vi "Copy (File).vi"(8 "error in (no error)":errorcluster, 9 "table":string, 10 "Path to spreadsheet":path, 11 "Data.PGSQL":refnum<class "LV-Data.PGSQL.lvclass">) -> (0 "error out":errorcluster, 3 "Data.PGSQL out":refnum<class "LV-Data.PGSQL.lvclass">)   [LabVIEW 2019, in "LV-Data.PGSQL.lvclass"]
uses:
  LV-Data.PGSQL.lvclass
  <vilib>/JDP Science/PostgreSQL Library/Connection/PQ Connection.lvclass
  LV-Data.PGSQL.lvclass/LV-Data.PGSQL.ctl
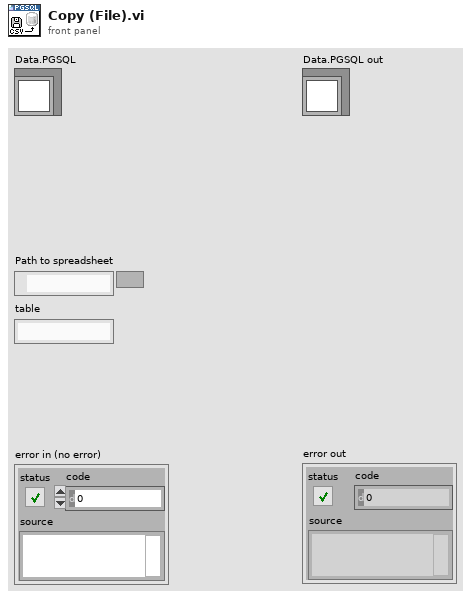
[diagram p1: front panel]
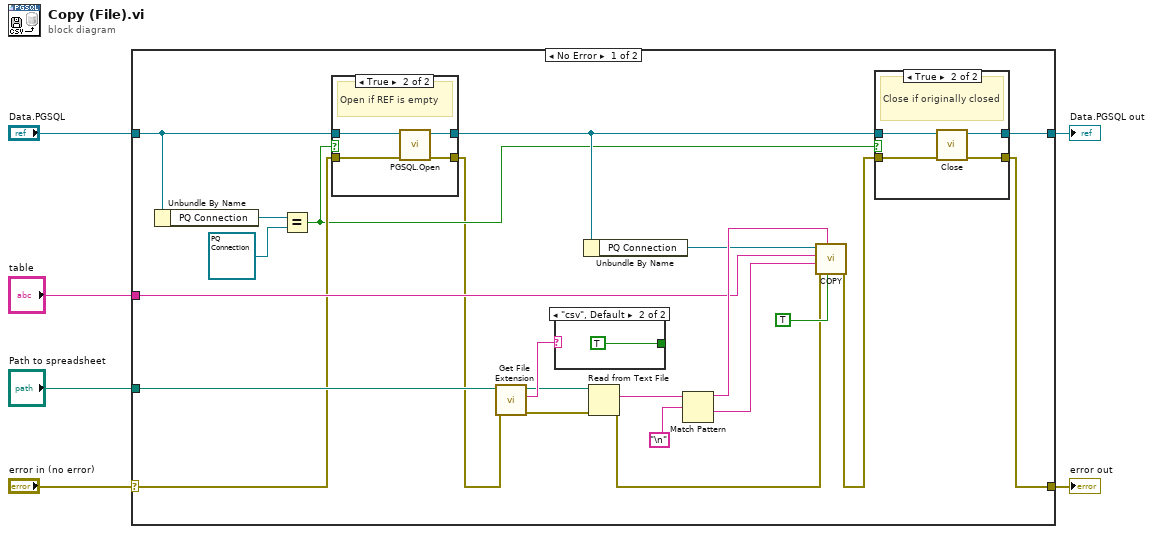
[diagram p0: block diagram]
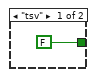
[diagram p3: hidden frame]
diagram:
  n1 = case shown="No Error" "error in (no error)" {
    selector: "error in (no error)" -> [w9 w44]
    tunnel: "table" -> [w17 _]
    tunnel: "Path to spreadsheet" -> [w23 _]
    tunnel: "Data.PGSQL" -> [w10 w43]
    tunnel: [w15 w44] -> w3
    tunnel: [w16 w43] -> w1
    frame No Error {
      n2 = Unbundle By Name(w10) -> ("PQ Connection"=w12:refnum<class "PQ Connection.lvclass">)
      n3 = Equal?(x=w12, y=refnum<class "PQ Connection.lvclass"> refnum ("PQ Connection")) -> (x = y?=w8:bool)
      n4 = case shown="True" w8 {
        tunnel: w10 -> [w29 w32]
        tunnel: [w30 w34] -> w7
        tunnel: w9 -> [w30 w33]
        tunnel: [w29 w31] -> w11
        frame False {
        }
        frame True {
          # "Open if REF is empty"
          n5 = call "PGSQL.Open.vi"("error in (no error)"=w33, "Data.PG in"=w32) -> ("error out"=w34:errorcluster, "Data.PG out"=w31:refnum<class "LV-Data.PGSQL.lvclass">)  [unwired: 8 in]
        }
      }
      n6 = call <vilib>:"Get File Extension.vi"("error in (no error)"=w7, "file"=w23) -> ("error out"=w24:errorcluster, "lowercase file extension"=w26:string, "dup file"=w25:path)  [unwired: 5 in, 2 out]
      n7 = case shown="\"csv\", Default" w26 {
        tunnel: [FALSE TRUE] -> _
        frame "tsv" {
        }
        frame "csv", Default {
        }
      }
      n8 = Unbundle By Name(w11) -> ("PQ Connection"=w18:refnum<class "PQ Connection.lvclass">)
      n9 = Read from Text File(file (use dialog)=w25, error in=w24) -> (text=w28:string, error out=w19:errorcluster)  [unwired: 2 in, 2 out]
      n10 = Match Pattern(string=w28, regular expression="\n") -> (before substring=w20:string, after substring=w21:string)  [unwired: 1 in, 2 out]
      n11 = call <vilib>:"COPY.vi"("CSV?"=TRUE, "column name(s) (empty=ALL)"=w20, "error in (no error)"=w19, "buffer"=w21, "table name"=w17, "PQ Connection in"=w18) -> ("error out"=w14:errorcluster)  [unwired: 4 in, 1 out]
      n12 = case shown="True" w8 {
        tunnel: w11 -> [w37 w42]
        tunnel: w14 -> [w38 w41]
        tunnel: [w38 w40] -> w15
        tunnel: [w37 w39] -> w16
        frame False {
          # "Do not close if closed wasn't before"
        }
        frame True {
          # "Close if originally closed"
          n13 = call-dynamic "Close.vi"("error in (no error)"=w41, "Data.PG in"=w42) -> ("error out"=w40:errorcluster, "Data.PG out"=w39:refnum<class "LV-Data.PGSQL.lvclass">)  [unwired: 8 in]
        }
      }
    }
    frame Error {
    }
  }
  "error out" <- w3
  "Data.PGSQL out" <- w1
